vi "Get Config@69.vi"(0 "Sequence path":path=path "C:/ModisEdge/Scope/Test Sequence/ModisEdge.ini", 7 "File":string="ModisEdge.ini") -> (1 "Headers Path":path=path "C:/ModisEdge/Scope/Test Sequence/Headers_ModisEdge.ini", 2 "FixtureID":string="MEScope_Fixture1", 3 "StopTestOnFailure":bool=TRUE, 4 "StationID":string="TSNAFT202", 6 "Test Report Path":path=path "C:/Snap-On/ModisEdge_Scope", 8 "DAQ DEVICE NAME":string="Dev5", 10 "WriteTheHeaders":bool, 14 "UUT_COM":u32=5, 15 "error out":errorcluster)   [LabVIEW 2015]
uses:
  <vilib>/Utility/config.llb/Read Key (Boolean).vi
  <vilib>/Utility/config.llb/Read Key (String).vi
  <vilib>/Utility/config.llb/Read Key (Path).vi
  <vilib>/Utility/config.llb/Read Key (U32).vi
  <vilib>/Utility/config.llb/NI_LVConfig.lvlib
panel:
  out "appended path":path=path "C:/ModisEdge/Scope/Test Sequence/ModisEdge.ini"
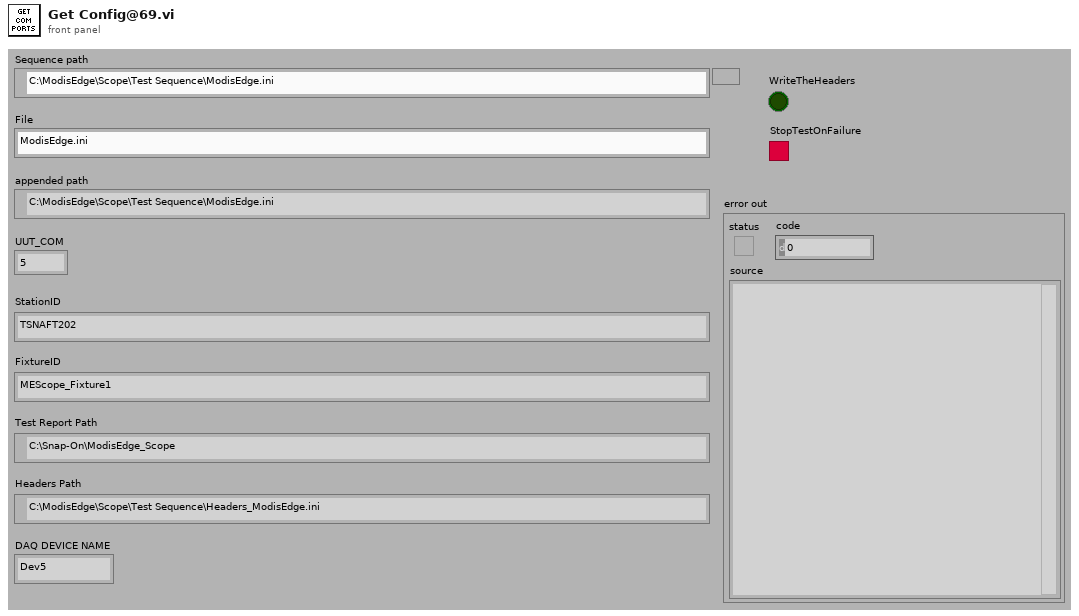
[diagram p1: front panel]
types:
  T1 = typedef "NI_LVConfig.lvlib/Config Data RefNum.ctl" = refnum<k1>
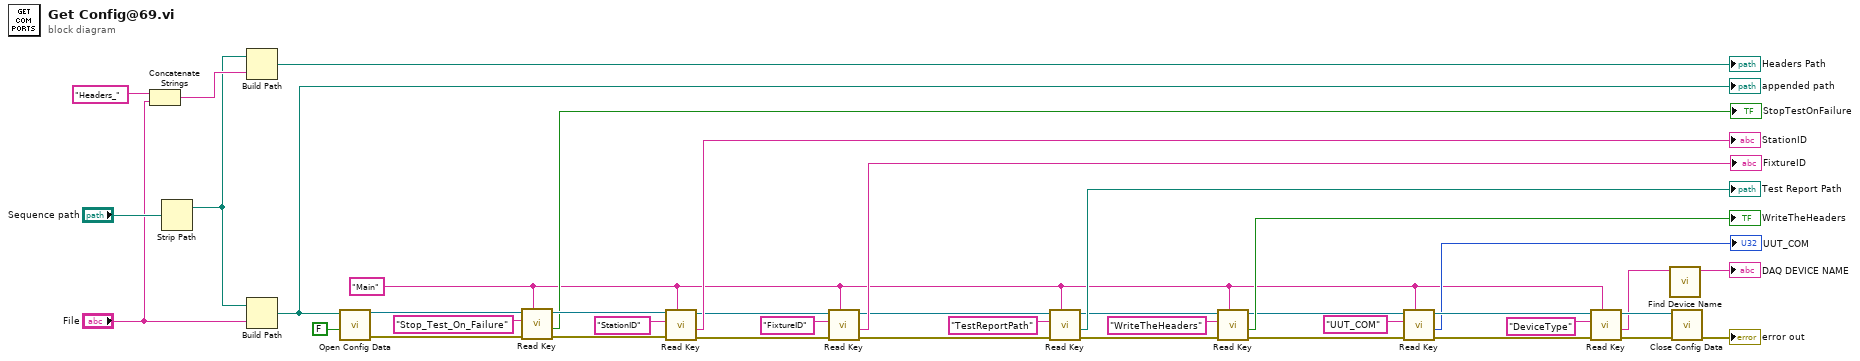
[diagram p0: block diagram]
diagram:
  w1 = "Main" ("section")
  n1 = Concatenate Strings("Headers_", "File") -> (w21:string)
  n2 = Strip Path(path="Sequence path") -> (stripped path=w20:path)  [unwired: 1 out]
  n3 = Build Path(base path=w20, name or relative path=w21) -> (appended path=→"Headers Path":path)
  n4 = Build Path(base path=w20, name or relative path="File") -> (appended path=w18:path)
  "appended path" <- w18
  n5 = call <vilib>:"Open Config Data.vi"("create file if necessary (T)"=FALSE, "configuration file path"=w18) -> ("error out"=w15:errorcluster, "refnum"=w16:T1)  [unwired: 7 in, 1 out]
  n6 = call-poly <vilib>:"Read Key.vi"("section"=w1, "error in (no error)"=w15, "key"="Stop_Test_On_Failure", "refnum"=w16) -> ("error out"=w14:errorcluster, "value"=→"StopTestOnFailure":bool, "refnum out"=w17:T1)  [unwired: 4 in, 1 out]
  n7 = call-poly <vilib>:"Read Key.vi"("section"=w1, "error in (no error)"=w14, "key"="StationID", "refnum"=w17) -> ("error out"=w6:errorcluster, "value"=→"StationID":string, "refnum out"=w2:T1)  [unwired: 4 in, 1 out]
  n8 = call-poly <vilib>:"Read Key.vi"("section"=w1, "error in (no error)"=w6, "key"="FixtureID", "refnum"=w2) -> ("error out"=w5:errorcluster, "value"=→"FixtureID":string, "refnum out"=w3:T1)  [unwired: 4 in, 1 out]
  n9 = call-poly <vilib>:"Read Key.vi"("section"=w1, "error in (no error)"=w5, "key"="TestReportPath", "refnum"=w3) -> ("error out"=w33:errorcluster, "value"=→"Test Report Path":path, "refnum out"=w32:T1)  [unwired: 4 in, 1 out]
  n10 = call-poly <vilib>:"Read Key.vi"("section"=w1, "error in (no error)"=w33, "key"="WriteTheHeaders", "refnum"=w32) -> ("error out"=w27:errorcluster, "value"=→"WriteTheHeaders":bool, "refnum out"=w11:T1)  [unwired: 4 in, 1 out]
  n11 = call-poly <vilib>:"Read Key.vi"("section"=w1, "error in (no error)"=w27, "key"="UUT_COM", "refnum"=w11) -> ("error out"=w12:errorcluster, "value"=→"UUT_COM":u32, "refnum out"=w10:T1)  [unwired: 4 in, 1 out]
  n12 = call-poly <vilib>:"Read Key.vi"("section"=w1, "error in (no error)"=w12, "key"="DeviceType", "refnum"=w10) -> ("error out"=w26:errorcluster, "value"=w24:string, "refnum out"=w25:T1)  [unwired: 4 in, 1 out]
  n13 = call "Find Device Name.vi"("Device Type"=w24) -> ("Device Name"=→"DAQ DEVICE NAME":string)  [unwired: 10 in]
  n14 = call <vilib>:"Close Config Data.vi"("error in (no error)"=w26, "refnum"=w25) -> ("error out"=→"error out":errorcluster)  [unwired: 8 in, 1 out]
